vi "OCR_Determine row type from colors.vi"(6 "Frame":T2, 8 "Error":errorcluster, 9 "Count":u32[](array[numeric]), 10 "Sorted By Quantity":u32[](array[colorbox]), 11 "Color List":u32[](array[colorbox])) -> (0 "Error Out":errorcluster, 2 "Highest Quanity Colors Out":T1={"BG"=239, "FG"=65793}, 3 "Type Out":T3)   [LabVIEW 2009]
doc: "Determines the row type of the color list"
uses:
  Controls/Enum/ENUM_Line Letter Type.ctl
  Controls/Enum/ENUM_Frame Template Select.ctl
  Controls/Cluster/Cluster_Text Color Set.ctl
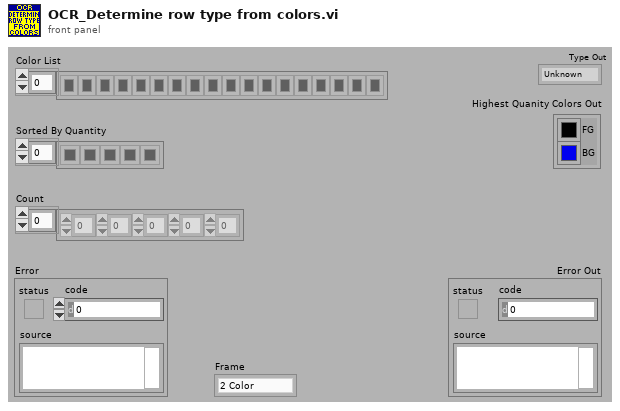
[diagram p1: front panel]
types:
  T1 = typedef "Cluster_Text Color Set.ctl" = cluster{"BG":u32, "FG":u32}
  T2 = typedef "ENUM_Frame Template Select.ctl" = enum16{"2 Color", "5 Color"}
  T3 = typedef "ENUM_Line Letter Type.ctl" = enum16{"Unknown", "Letter", "Seperator", "Seperator or Letter"}
  T4 = cluster{"Sorted By Quantity[0]":u32, "Sorted By Quantity[1]":u32}
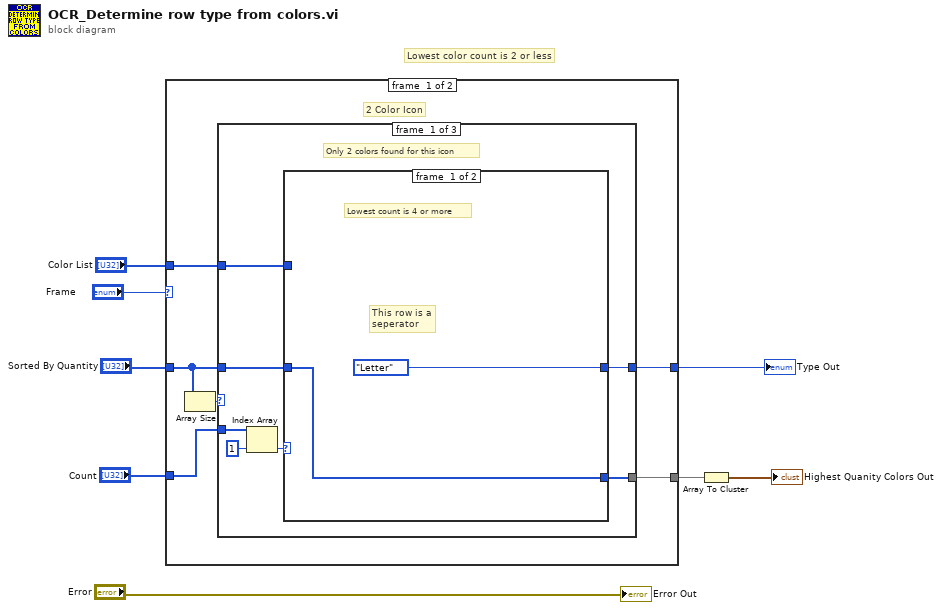
[diagram p0: block diagram]
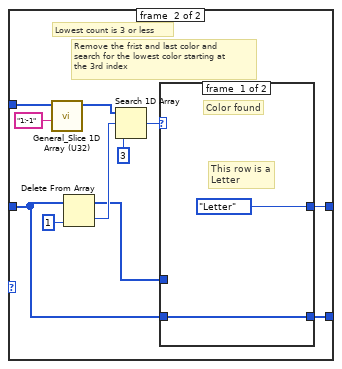
[diagram p2: hidden frame]
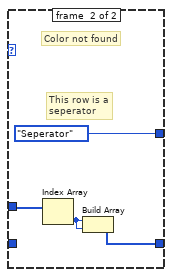
[diagram p3: hidden frame]
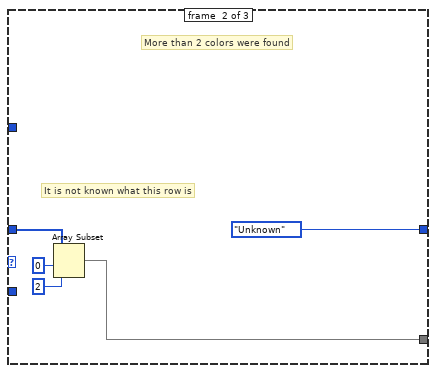
[diagram p4: hidden frame]
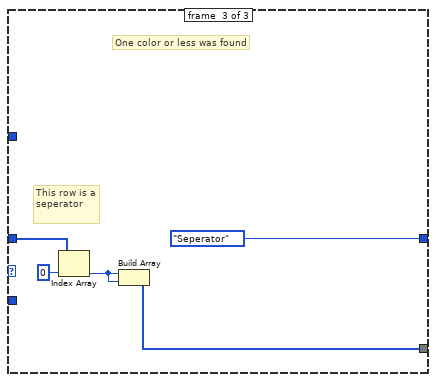
[diagram p5: hidden frame]
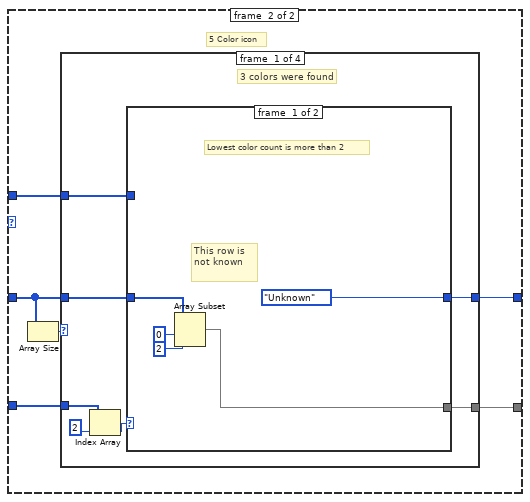
[diagram p6: hidden frame]
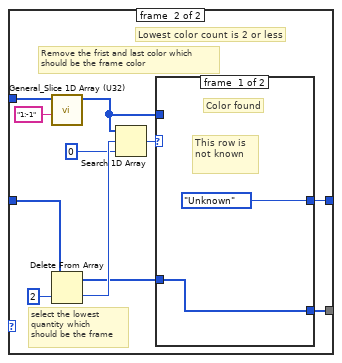
[diagram p7: hidden frame]
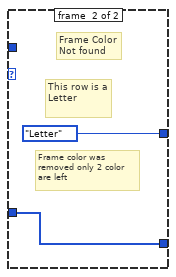
[diagram p8: hidden frame]
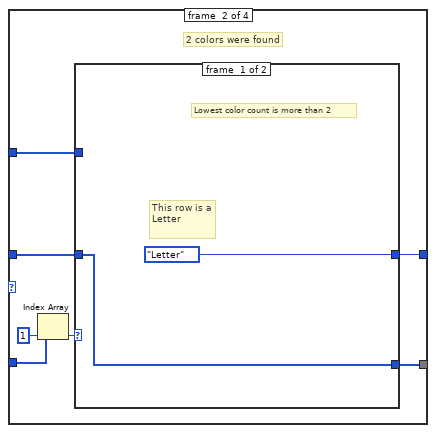
[diagram p9: hidden frame]
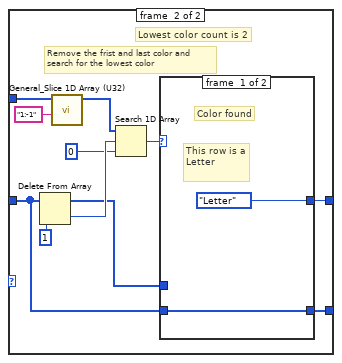
[diagram p10: hidden frame]
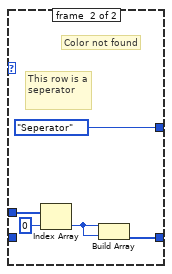
[diagram p11: hidden frame]
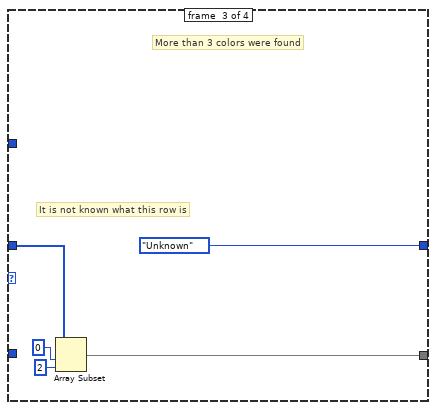
[diagram p12: hidden frame]
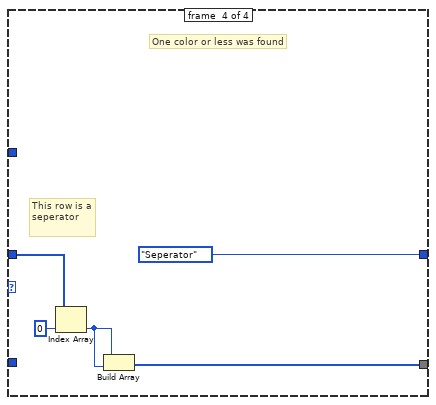
[diagram p13: hidden frame]
diagram:
  # "Lowest color count is 2 or less"
  n1 = case shown="\"5 Color\"" "Frame" {
    tunnel: [w14 w56] -> w7
    tunnel: "Sorted By Quantity" -> [w13 w55]
    tunnel: "Count" -> [w11 w53]
    tunnel: "Color List" -> [w10 w52]
    tunnel: [w9 w51] -> w2
    frame #0 {
      # "2 Color Icon"
      n2 = Array Size(array=w13) -> (size(s)=w12:i32)
      n3 = case shown="2" w12 {
        tunnel: [w21 ENUM_Line_Letter_Type."Unknown" ("Type Out") ENUM_Line_Letter_Type."Seperator" ("Type Out")] -> w14
        tunnel: w13 -> [w17 w44 w49]
        tunnel: w11 -> [w20 _ _]
        tunnel: w10 -> [w16 _ _]
        tunnel: [w15 w41 w46] -> w9
        frame #0 {
          # "Only 2 colors found for this icon"
          n4 = Index Array(array=w20, index=1) -> (element=w18:u32)
          n5 = case shown="Default" w18 {
            tunnel: [ENUM_Line_Letter_Type."Letter" ("Type Out") w34] -> w21
            tunnel: w16 -> [_ w28]
            tunnel: w17 -> [w22 w25]
            tunnel: [w22 w26] -> w15
            frame #0 {
              # "This row is a \nseperator"
              # "Lowest count is 4 or more"
            }
            frame #1 {
              # "Lowest count is 3 or less"
              # "Remove the frist and last color and\nsearch for the lowest color starting at\nthe 3rd index"
              n6 = call "General_Slice 1D Array (U32).vi"("Slice"="1:-1" ("slice"), "Array"=w28) -> ("Array Out"=w27:u32[])  [unwired: 8 in, 1 out]
              n7 = Delete From Array(array=w25, index=1) -> (deleted portion=w32:u32, array with subset deleted=w24:u32[])  [unwired: 1 in]
              n8 = Search 1D Array(1D array=w27, element=w32, start index (0)=3) -> (index of element=w31:i32)
              n9 = case shown="-1" w31 {
                tunnel: [ENUM_Line_Letter_Type."Letter" ("Type Out") ENUM_Line_Letter_Type."Seperator" ("Type Out")] -> w34
                tunnel: w25 -> [w35 _]
                tunnel: [w35 w37] -> w26
                tunnel: w24 -> [_ w39]
                frame #0 {
                  # "This row is a \nLetter"
                  # "Color found"
                }
                frame #1 {
                  # "This row is a \nseperator"
                  # "Color not found"
                  n10 = Index Array(array=w39) -> (element=w38:u32)  [unwired: 1 in]
                  n11 = Build Array(w38, w38) -> (w37:u32[])
                }
              }
            }
          }
        }
        frame #1 {
          # "It is not known what this row is"
          # "More than 2 colors were found"
          n12 = Array Subset(array=w44, index=0, length=2) -> (w41:u32[])
        }
        frame #2 {
          # "This row is a \nseperator"
          # "One color or less was found"
          n13 = Index Array(array=w49, index=0) -> (element=w47:u32)
          n14 = Build Array(w47, w47) -> (w46:u32[])
        }
      }
    }
    frame #1 {
      # "5 Color icon"
      n15 = Array Size(array=w55) -> (size(s)=w54:i32)
      n16 = case shown="2" w54 {
        tunnel: [w63 w90 ENUM_Line_Letter_Type."Unknown" ("Type Out") ENUM_Line_Letter_Type."Seperator" ("Type Out")] -> w56
        tunnel: w55 -> [w60 w86 w114 w119]
        tunnel: w53 -> [w62 w89 _ _]
        tunnel: w52 -> [w59 w85 _ _]
        tunnel: [w58 w84 w113 w116] -> w51
        frame #0 {
          # "3 colors were found"
          n17 = Index Array(array=w62, index=2) -> (element=w61:u32)
          n18 = case shown="Default" w61 {
            tunnel: [ENUM_Line_Letter_Type."Unknown" ("Type Out") w79] -> w63
            tunnel: w59 -> [_ w72]
            tunnel: w60 -> [w67 w78]
            tunnel: [w64 w70] -> w58
            frame #0 {
              # "Lowest color count is more than 2"
              # "This row is not known"
              n19 = Array Subset(array=w67, index=0, length=2) -> (w64:u32[])
            }
            frame #1 {
              # "select the lowest \nquantity which \nshould be the frame"
              # "Remove the frist and last color which\nshould be the frame color"
              # "Lowest color count is 2 or less"
              n20 = call "General_Slice 1D Array (U32).vi"("Slice"="1:-1" ("slice"), "Array"=w72) -> ("Array Out"=w71:u32[])  [unwired: 8 in, 1 out]
              n21 = Delete From Array(array=w78, index=2) -> (deleted portion=w76:u32, array with subset deleted=w69:u32[])  [unwired: 1 in]
              n22 = Search 1D Array(1D array=w71, element=w76, start index (0)=0) -> (index of element=w75:i32)
              n23 = case shown="-1" w75 {
                tunnel: [ENUM_Line_Letter_Type."Unknown" ("Type Out") ENUM_Line_Letter_Type."Letter" ("Type Out")] -> w79
                tunnel: w71 -> [_ _]
                tunnel: [w80 w82] -> w70
                tunnel: w69 -> [w80 w82]
                frame #0 {
                  # "This row is not known"
                  # "Color found"
                }
                frame #1 {
                  # "Frame color was \nremoved only 2 color\nare left"
                  # "This row is a \nLetter"
                  # "Frame Color \nNot found"
                }
              }
            }
          }
        }
        frame #1 {
          # "2 colors were found"
          n24 = Index Array(array=w89, index=1) -> (element=w87:u32)
          n25 = case shown="..2" w87 {
            tunnel: [ENUM_Line_Letter_Type."Letter" ("Type Out") w103] -> w90
            tunnel: w85 -> [_ w97]
            tunnel: w86 -> [w91 w93]
            tunnel: [w91 w94] -> w84
            frame #0 {
              # "This row is a \nLetter"
              # "Lowest color count is more than 2"
            }
            frame #1 {
              # "Remove the frist and last color and\nsearch for the lowest color"
              # "Lowest color count is 2"
              n26 = Delete From Array(array=w93, index=1) -> (deleted portion=w101:u32, array with subset deleted=w95:u32[])  [unwired: 1 in]
              n27 = call "General_Slice 1D Array (U32).vi"("Slice"="1:-1" ("slice"), "Array"=w97) -> ("Array Out"=w96:u32[])  [unwired: 8 in, 1 out]
              n28 = Search 1D Array(1D array=w96, element=w101, start index (0)=0) -> (index of element=w100:i32)
              n29 = case shown="Default" w100 {
                tunnel: [ENUM_Line_Letter_Type."Letter" ("Type Out") ENUM_Line_Letter_Type."Seperator" ("Type Out")] -> w103
                tunnel: w95 -> [_ w109]
                tunnel: [w104 w106] -> w94
                tunnel: w93 -> [w104 _]
                frame #0 {
                  # "This row is a \nLetter"
                  # "Color found"
                }
                frame #1 {
                  # "Color not found"
                  # "This row is a \nseperator"
                  n30 = Index Array(array=w109, index=0) -> (element=w107:u32)
                  n31 = Build Array(w107, w107) -> (w106:u32[])
                }
              }
            }
          }
        }
        frame #2 {
          # "It is not known what this row is"
          # "More than 3 colors were found"
          n32 = Array Subset(array=w114, index=0, length=2) -> (w113:u32[])
        }
        frame #3 {
          # "This row is a \nseperator"
          # "One color or less was found"
          n33 = Index Array(array=w119, index=0) -> (element=w117:u32)
          n34 = Build Array(w117, w117) -> (w116:u32[])
        }
      }
    }
  }
  "Type Out" <- w7
  n35 = Array To Cluster(array=w2) -> (cluster=→"Highest Quanity Colors Out":T4)
  "Error Out" <- "Error"
